vi "Analysis_Lin_input.vi"() -> ()   [LabVIEW 2010]
doc: "Use this template to generate a signal, analyze the signal, and display the result. You can use this template with the exercises in the Getting Started with LabVIEW manual.\nNote: LabVIEW enables automatic error handling by default for VIs you create from this template."
uses:
  <vilib>/measure/maspectr.llb/FFT Power Spectrum and PSD for 1 Chan.vi
  <vilib>/measure/NI_MAPro.lvlib
panel:
  out "max":i32
  out "df_X":dbl
  out "FFT from X":cluster{"f0":dbl, "df":dbl, "magnitude":dbl[]}(graph)
  out "magnitude_X":dbl[](array[numeric])
  out "f0_X":dbl
  out "Signal from X":waveform(dbl)(graph)
  in  "stop":bool
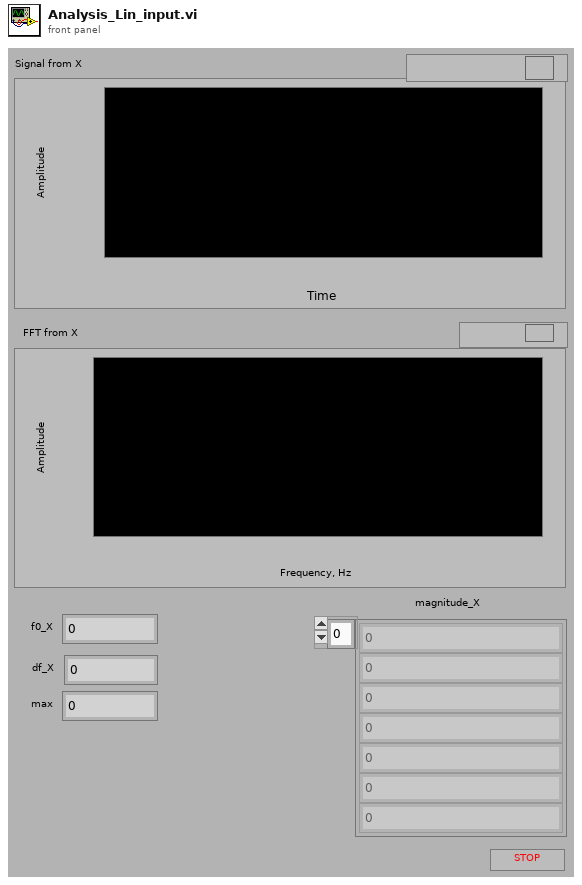
[diagram p1: front panel]
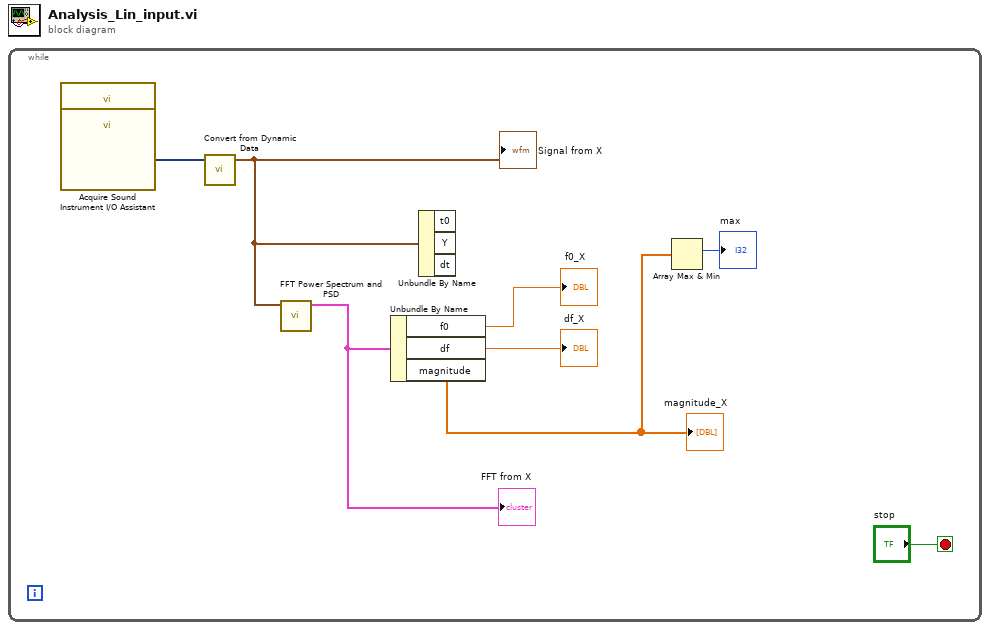
[diagram p0: block diagram]
diagram:
  n1 = while {
    stop <- "stop" stop-if-true
    n2 = call "Acquire Sound"() -> ("Data"=w4:dynamicdata)  [unwired: 18 in, 1 out]
    n3 = call "Instrument I/O Assistant"() -> ()  [unwired: 28 in]
    n4 = call "Convert from Dynamic Data"("Dynamic Data Type"=w4) -> ("Waveform"=w7:waveform(dbl))  [unwired: 3 in]
    "Signal from X" <- w7
    n5 = call-poly <vilib>:"FFT Power Spectrum and PSD.vi"("time signal"=w7) -> ("Power Spectrum / PSD"=w5:cluster{"f0":dbl, "df":dbl, "magnitude":dbl[]})  [unwired: 7 in, 3 out]
    "FFT from X" <- w5
    n6 = Unbundle By Name(w5) -> ("f0"=→"f0_X":dbl, "df"=→"df_X":dbl, "magnitude"=w1:dbl[])
    "magnitude_X" <- w1
    n7 = Unbundle By Name(w7) -> ()  [unwired: 3 out]
    n8 = Array Max & Min(array=w1) -> (max index (indices)=→"max":i32)  [unwired: 3 out]
  }
